vi "Initialise on load.vi"(11 "OldVal":path) -> ()   [LabVIEW 2020]
uses:
  Experiment header interface/Typedefs/Header file interface module functions enum.ctl
  Global variables/gl_Functional Imaging-Global variables.vi
  Experiment header interface/Typedefs/Header file type enum.ctl
panel:
  in  "error in":errorcluster
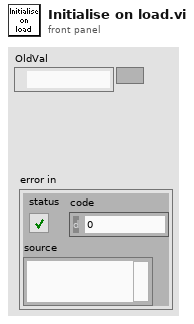
[diagram p1: front panel]
types:
  T1 = typedef "Functional Imging UI Refs.ctl" = cluster{"Menu ref":refnum<k9>, "Image control":refnum<vi>, "VI ref":refnum<vi>, "XGrapher":refnum<vi>, "Smoothing":refnum<vi>, "POI Averaging":refnum<vi>, "Normalize":refnum<vi>, "POI data points in each trial":refnum<vi>, "Channel":refnum<vi>, "Experiment data folder path":refnum<vi>, "[ROI vis]":refnum<vi>, "[Groups] visbl":T2, "Group Name":refnum<vi>, "POI index":refnum<vi>, "Trial No.":refnum<vi>, "Intensity Zoom":refnum<vi>, "Trial Cursor Enabled":refnum<vi>, "Number of Trials (ind 1)":refnum<vi>, "Number of Trials (ind 2)":refnum<vi>, "MiniScans Available":refnum<vi>, "POI Available":refnum<vi>, "Defer graph updates":refnum<vi>, "Waveform selector":refnum<vi>, "#of selected POI":refnum<vi>, "#of selected MiniScans":refnum<vi>, "#of selected groups":refnum<vi>, "Max Z-Projection":refnum<vi>, "Z-Plane Selector":refnum<vi>, "Index of miniscan point to visualise":refnum<vi>, "ROI vis. mode":refnum<vi>, "Total # of points":refnum<vi>, "Index of group clicked on":refnum<vi>, "Pane 1":refnum<vi>, "Pane 2":refnum<vi>, "Pane 3":refnum<vi>, "Pane 4":refnum<vi>, "Pane 5":refnum<vi>, "Pane 6":refnum<vi>, "Deselect all ROI":refnum<vi>, "Deselect all groups":refnum<vi>}
  T2 = typedef "Groups array referecne.ctl" = refnum<vi>
  T3 = typedef "Header file interface module functions enum.ctl" = enum16{"Load experiment header file", "Save experiment header file", "Clear stored values", "Read stored values", "Update specific value in memory", "Update values in memory"}
  T4 = typedef "Header file type enum.ctl" = enum16{"All parameters", "Params for funct acq w ROI or mscn", "Params for funct acq w rectangles", "Live imaging header parameters", "AOL Parameters"}
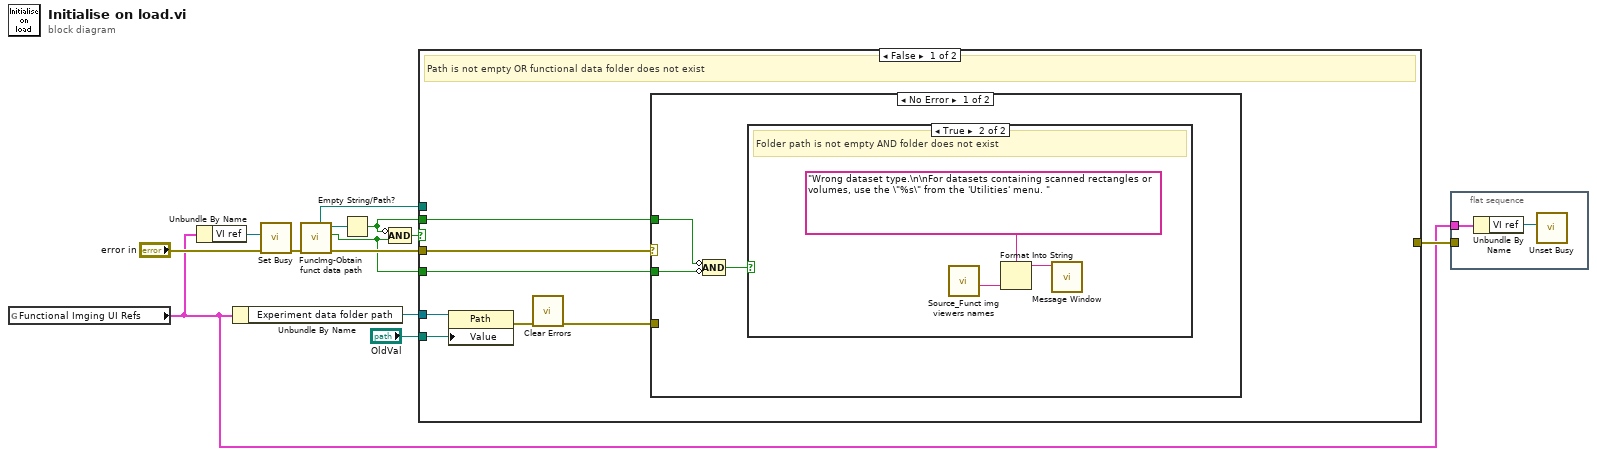
[diagram p0: block diagram]
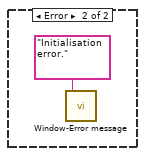
[diagram p3: hidden frame]
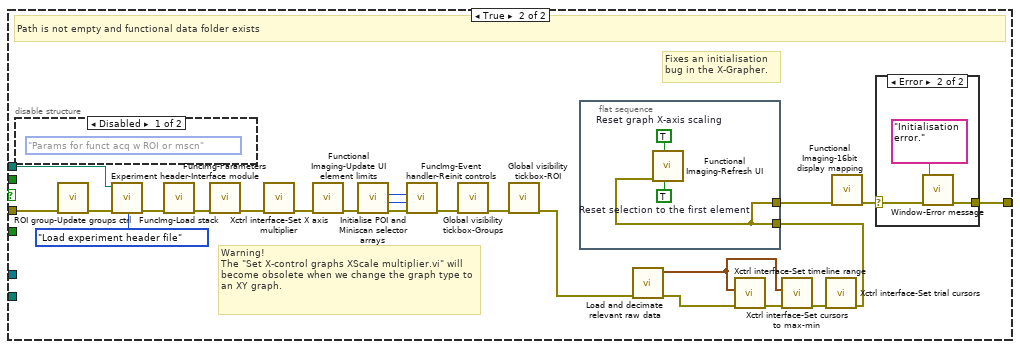
[diagram p4: hidden frame]
diagram:
  n1 = global read "gl_Functional Imaging-Global variables.vi" "Functional Imging UI Refs"() -> (w1:T1)
  n2 = Unbundle By Name(w1) -> ("VI ref"=w5:refnum<vi>)
  n3 = Unbundle By Name(w1) -> ("Experiment data folder path"=w6:refnum<vi>)
  n4 = call <vilib>:"Set Busy.vi"("error in (no error)"="error in", "VI reference (current VI)"=w5) -> ("error out"=w2:errorcluster)  [unwired: 8 in, 1 out]
  n5 = call "FuncImg-Obtain funct data path.vi"("error in"=w2) -> ("error out"=w13:errorcluster, "file or folder exists?"=w8:bool, "Functional data folder path"=w9:path, "Experiment data folder path"=w10:path)  [unwired: 6 in, 1 out]
  n6 = Empty String/Path?(string/path=w9) -> (empty?=w11:bool)
  n7 = Compound Arithmetic op=AND(invert w11, w8) -> (w12:bool)
  n8 = case shown="False" w12 {
    tunnel: w10 -> [_ w42]
    tunnel: w13 -> [w20 w38]
    tunnel: w8 -> [w19 _]
    tunnel: w11 -> [w18 _]
    tunnel: w6 -> [w17 _]
    tunnel: "OldVal" -> [w14 _]
    tunnel: [_ w28] -> w4
    frame False {
      # "Path is not empty OR functional data folder does not exist"
      n9 = property class="Path"(reference=w17, "Value"=w14) -> (error out=w16:errorcluster)  [unwired: 1 in, 1 out]
      n10 = call <vilib>:"Clear Errors.vi"("error in (no error)"=w16) -> ("error out"=w15:errorcluster)  [unwired: 5 in, 1 out]
      n11 = case shown="No Error" w20 {
        tunnel: w19 -> [w22 _]
        tunnel: w18 -> [w23 _]
        tunnel: w15 -> [_ _]
        frame No Error {
          n12 = Compound Arithmetic op=AND(invert w23, invert w22) -> (w21:bool)
          n13 = case shown="True" w21 {
            frame False {
              # "Path is empty or folder does not exist"
            }
            frame True {
              # "Folder path is not empty AND folder does not exist"
              n14 = call "Source_Funct img viewers names.vi"() -> ("Name string: Functional imaging viewer (Rectangles)"=w25:string)  [unwired: 10 in, 1 out]
              n15 = Format Into String(format string="Wrong dataset type.\n\nFor datasets containing scanned rectangles or volumes, use the \"%s\" from the 'Utilities' menu. " ("Message"), w25) -> (resulting string=w24:string)  [unwired: 2 in, 1 out]
              n16 = call "Message Window.vi"("Message string"=w24) -> ()  [unwired: 10 in, 1 out]
            }
          }
        }
        frame Error {
          n17 = call "Window-Error message.vi"("Message"="Initialisation error.") -> ()  [unwired: 10 in, 1 out]
        }
      }
    }
    frame True {
      # "Fixes an initialisation \nbug in the X-Grapher."
      # "Warning!\nThe \"Set X-control graphs XScale multiplier.vi\" will become obsolete when we change the graph type to an XY graph."
      # "Path is not empty and functional data folder exists"
      n18 = disable-structure shown="Disabled" {
        frame Disabled {
          (unwired) Header_file_type_enum."Params for funct acq w ROI or mscn" ("Header file type")
        }
        frame Enabled {
        }
      }
      n19 = call "ROI group-Update groups ctrl.vi"("error in (no error)"=w38) -> ("error out"=w39:errorcluster)  [unwired: 10 in]
      n20 = call "Experiment header-Interface module.vi"("error in (no error)"=w39, "Function"=Header_file_interface_module_functions_enum."Load experiment header file", "Experiment data folder path"=w42) -> ("error out"=w48:errorcluster)  [unwired: 7 in, 1 out]
      n21 = call "FuncImg-Load stack.vi"("Error In"=w48) -> ("Error Out"=w49:errorcluster)  [unwired: 11 in, 3 out]
      n22 = call "FuncImg-Parameters.vi"("Error In"=w49) -> ("Error Out"=w46:errorcluster)  [unwired: 14 in]
      n23 = call "Xctrl interface-Set X axis multiplier.vi"("error in (no error)"=w46) -> ("error out"=w45:errorcluster)  [unwired: 10 in]
      n24 = call "Functional Imaging-Update UI element limits.vi"("error in (no error)"=w45) -> ("error out"=w50:errorcluster)  [unwired: 10 in]
      n25 = call "Initialise POI and Miniscan selector arrays.vi"("error in (no error)"=w50) -> ("error out"=w37:errorcluster, "Number of POI"=w41:i32, "Number of Miniscans"=w40:i32)  [unwired: 7 in, 1 out]
      n26 = call "FuncImg-Event handler-Reinit controls.vi"("error in"=w37, "Number of POI"=w41, "Number of Miniscans"=w40) -> ("Error out"=w36:errorcluster)  [unwired: 8 in]
      n27 = call "Global visibility tickbox-Groups.vi"("error in (no error)"=w36) -> ("error out"=w35:errorcluster)  [unwired: 10 in]
      n28 = call "Global visibility tickbox-ROI.vi"("error in (no error)"=w35) -> ("error out"=w29:errorcluster)  [unwired: 10 in]
      n29 = flat-sequence {
        tunnel: w34 -> [w55]
        tunnel: [w55] -> w33
        frame #0 {
          w56 = TRUE  # Reset selection to the first element
          w57 = TRUE  # Reset graph X-axis scaling
          n30 = call "Functional Imaging-Refresh UI.vi"("Select the first element"=w56, "Reset graph X-axis scaling (F)"=w57, "error in (no error)"=w55) -> ()  [unwired: 9 in]
        }
      }
      n31 = call "Load and decimate relevant raw data.vi"("error in (no error)"=w29) -> ("error out"=w30:errorcluster, "X-axis max/min (across all loaded data types)"=w31:cluster{"X-axis max":dbl, "X-axis min":dbl})  [unwired: 7 in, 2 out]
      n32 = call "Xctrl interface-Set timeline range.vi"("error in (no error)"=w30, "X-axis max/min (across all loaded data types)"=w31) -> ("error out"=w44:errorcluster)  [unwired: 9 in]
      n33 = call "Xctrl interface-Set cursors to max-min.vi"("error in (no error)"=w44, "input cluster"=w31) -> ("error out"=w43:errorcluster)  [unwired: 9 in]
      n34 = call "Xctrl interface-Set trial cursors.vi"("error in (no error)"=w43) -> ("error out"=w34:errorcluster)  [unwired: 10 in]
      n35 = call "Functional Imaging-16bit display mapping.vi"("error in (no error)"=w33) -> ("error out"=w32:errorcluster)  [unwired: 10 in]
      n36 = case shown="Error" w32 {
        selector: w32 -> [w51 w54]
        tunnel: [w51 w52] -> w28
        frame No Error {
        }
        frame Error {
          n37 = call "Window-Error message.vi"("error in (no error)"=w54, "Message"="Initialisation error.") -> ("Error Out (no error)"=w52:errorcluster)  [unwired: 9 in]
        }
      }
    }
  }
  n38 = flat-sequence {
    tunnel: w4 -> [_]
    tunnel: w1 -> [w58]
    frame #0 {
      n39 = Unbundle By Name(w58) -> ("VI ref"=w59:refnum<vi>)
      n40 = call <vilib>:"Unset Busy.vi"("VI reference (current VI)"=w59) -> ()  [unwired: 10 in, 1 out]
    }
  }
